vi "Callback Change Direction.vi"(6 "Variant":variant, 8 "error in (no error)":errorcluster, 9 "old values":string[][](array[string]), 10 "object ref in":T1, 11 "Cluster":T2) -> (0 "error out":errorcluster)   [LabVIEW 2013, in "Modbus Module editor node.lvclass"]
uses:
  Modbus Module editor node.lvclass
  <vilib>/NI/DCAF Table API/Table Manager/Cell Change.ctl
  <vilib>/NI/DCAF Table API/Table Manager/object ref.ctl
  <vilib>/NI/DCAF/Tag Editor Core/Configuration Editor/Classes/Engine Parent/Engine Parent Editor Node.lvclass
  <vilib>/NI/DCAF/Tag Editor Core/Configuration Editor/Classes/Module editor node/module editor node.lvclass
  permissions.ctl
  <vilib>/NI/Tag Bus/tag/Data Type.ctl
  module/configuration/Modbus Module configuration.lvclass
  <vilib>/NI/Configuration Framework/serializable configuration/NISE_CEF_serializable configuration.lvclass/NISE_CEF_serializable configuration.ctl
  <vilib>/NI/Tag Bus Module Framework/channel/TBM channel.lvclass/TBM channel.ctl
  <vilib>/Utility/LVClass/Get LV Class Name.vi
  <vilib>/NI/Configuration Framework/error generator/NISE_error generator.vi
  <vilib>/NI/Module Execution Interface/Engine Configuration/engine configuration.lvclass
  <vilib>/NI/Configuration Framework/serializable configuration/NISE_CEF_serializable configuration.lvclass
  <vilib>/NI/DCAF Table API/Table Manager.lvlib
  <vilib>/NI/Tag Bus/tag/tag descriptor.lvclass
  <vilib>/NI/Tag Bus Module Framework/channel/TBM channel.lvclass
  <vilib>/NI/DCAF Table API/Table Manager/Table Manager.lvclass
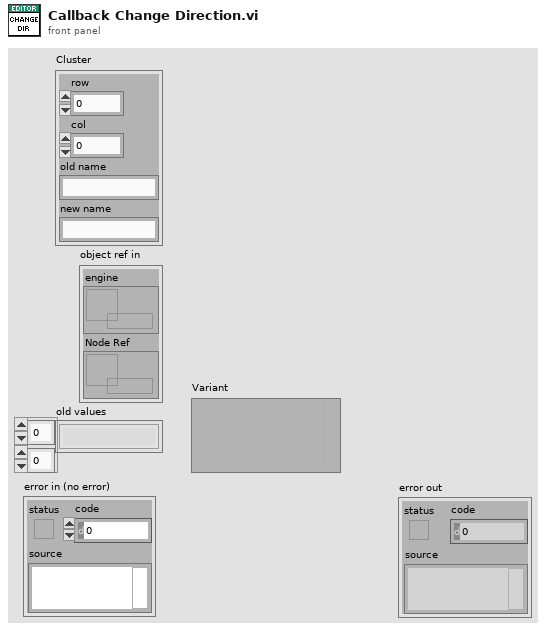
[diagram p1: front panel]
types:
  T1 = typedef "Table Manager.lvlib/Table Manager.lvclass/object ref.ctl" = cluster{"engine":refnum<data-value>, "Node Ref":refnum<data-value>}
  T2 = typedef "Table Manager.lvlib/Cell Change.ctl" = cluster{"row":i32, "col":i32, "old name":string, "new name":string}
  T3 = typedef "tag bus.lvlib/tag descriptor.lvclass/Data Type.ctl" = enum16{"Double", "Single", "I64", "I32", "I16", "I8", "U64", "U32", "U16", "U8", "Boolean", "String", "Array of Double", "Array of Single", "Array of I64", "Array of I32", "Array of I16", "Array of I8", "Array of U64", "Array of U32", "Array of U16", "Array of U8", "Array of Boolean", "Array of String"}
  T4 = typedef "Modbus Module editor node.lvclass/permissions.ctl" = enum32{"Read from MB", "Write to MB"}
  T5 = typedef "TBM channel.lvclass/channel classification.ctl" = enum16{"input data", "output data", "processing parameter", "processing result"}
  T6 = typedef "Modbus Module configuration.lvclass/Line.ctl" = refnum<class "Modbus Module Channel.lvclass">
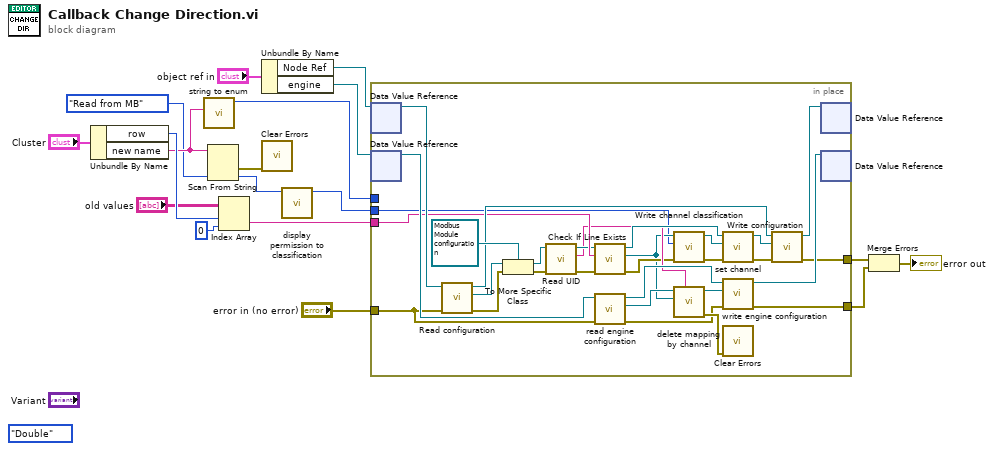
[diagram p0: block diagram]
diagram:
  (unwired) Data_Type."Double" ("data type")
  n1 = Unbundle By Name("Cluster") -> ("row"=w14:i32, "new name"=w5:string)
  n2 = call <vilib>:"string to enum.vi"("String"=w5) -> ("Value"=w6:i32)  [unwired: 9 in, 1 out]
  n3 = Scan From String(input string=w5, default 1=permissions."Read from MB" ("direction")) -> (error out=w3:errorcluster, output 1=w2:T4)  [unwired: 3 in, 2 out]
  n4 = Index Array(array="old values", index (row)=w14, index (col)=0 ("disabled index (col)")) -> (element=w12:string)
  n5 = Unbundle By Name("object ref in") -> ("Node Ref"=w16:refnum<data-value>, "engine"=w15:refnum<data-value>)
  n6 = call <vilib>:"Clear Errors.vi"("error in (no error)"=w3) -> ()  [unwired: 6 in, 1 out]
  n7 = call "display permission to classification.vi"("display permissions"=w2) -> ("channel classification"=w1:T5)  [unwired: 10 in]
  n8 = in-place {
    in-place-border: w12 -> [w40]
    in-place-border: "error in (no error)" -> [w25]
    in-place-border: [w27] -> w8
    in-place-border: [w26] -> w7
    in-place-border: w6 -> [_]
    in-place-border: w1 -> [w20]
    n9 = in-place-dvr #1(w16) -> (w45:refnum<class "module editor node.lvclass">)  [unwired: 1 out]
    n10 = in-place-dvr #2(w15) -> (w41:refnum<class "Engine Parent Editor Node.lvclass">)  [unwired: 1 out]
    n11 = call-dynamic "Read configuration.vi"("error in"=w25, "NISE_CEF_serializable node in"=w45) -> ("error out"=w28:errorcluster, "configuration"=w47:refnum<class "NISE_CEF_serializable configuration.lvclass">, "NISE_CEF_serializable node out"=w44:refnum<class "module editor node.lvclass">)  [unwired: 7 in]
    n12 = To More Specific Class(target class=refnum<class "Modbus Module configuration.lvclass"> refnum ("Modbus Slave configuration in"), reference=w47, error in=w28) -> (specific class reference=w37:refnum<class "Modbus Module configuration.lvclass">, error out=w31:errorcluster)
    n13 = call <vilib>:"Read UID.vi"("error in"=w31, "configuration in"=w37) -> ("error out"=w30:errorcluster, "instance id"=w35:string, "configuration out"=w36:refnum<class "Modbus Module configuration.lvclass">)  [unwired: 7 in]
    n14 = call "Check If Line Exists.vi"("error in (no error)"=w30, "Name to locate"=w40, "Modbus Slave configuration in"=w36) -> ("error out"=w22:errorcluster, "Line out"=w21:T6, "Modbus Slave configuration out"=w39:refnum<class "Modbus Module configuration.lvclass">)  [unwired: 4 in, 2 out]
    n15 = call <vilib>:"read engine configuration.vi"("error in"=w25, "Engine Parent Editor Node in"=w41) -> ("error out"=w24:errorcluster, "engine configuration"=w32:refnum<class "engine configuration.lvclass">, "Engine Parent Editor Node out"=w42:refnum<class "Engine Parent Editor Node.lvclass">)  [unwired: 7 in]
    n16 = call <vilib>:"Write channel classification.vi"("error in"=w22, "channel classification"=w20, "channel in"=w21) -> ("error out"=w23:errorcluster, "channel out"=w19:T6)  [unwired: 7 in]
    n17 = call <vilib>:"delete mapping by channel.vi"("owner ID"=w35, "channel"=w21, "engine configuration in"=w32) -> ("error out"=w34:errorcluster, "engine configuration out"=w33:refnum<class "engine configuration.lvclass">)  [unwired: 7 in]
    n18 = call "set channel.vi"("error in"=w23, "Modbus Module Channel.lvclass"=w19, "Modbus Slave configuration in"=w39) -> ("error out"=w29:errorcluster, "Modbus Slave configuration out"=w38:refnum<class "Modbus Module configuration.lvclass">)  [unwired: 7 in]
    n19 = call <vilib>:"write engine configuration.vi"("error in"=w24, "engine configuration"=w33, "Engine Parent Editor Node in"=w42) -> ("error out"=w27:errorcluster, "Engine Parent Editor Node out"=w43:refnum<class "Engine Parent Editor Node.lvclass">)  [unwired: 7 in]
    n20 = call <vilib>:"Clear Errors.vi"("error in (no error)"=w34) -> ()  [unwired: 6 in, 1 out]
    n21 = call-dynamic "Write configuration.vi"("error in"=w29, "configuration"=w38, "NISE_CEF_serializable node in"=w44) -> ("error out"=w26:errorcluster, "NISE_CEF_serializable node out"=w46:refnum<class "module editor node.lvclass">)  [unwired: 7 in]
    n22 = in-place-dvr #1(w46) -> ()  [unwired: 2 out]
    n23 = in-place-dvr #2(w43) -> ()  [unwired: 2 out]
  }
  n24 = Merge Errors(w7, w8) -> (→"error out":errorcluster)
